vi "Initial Signal Processing.vi"(8 "error in":errorcluster, 11 "AI Ref In":T1) -> (0 "error out":errorcluster, 1 "max value":dbl, 2 "Wheeze?":bool[](array[boolean]), 3 "AI Ref Out 2":T1)   [LabVIEW 2019]
doc: "The myRIO Project template acquires acceleration data from the onboard accelerometer and displays the changes of acceleration values in a waveform chart."
uses:
  <vilib>/myRIO/Instrument Drivers/Onboard IO/AI/typedefs/AI Reference.ctl
  <vilib>/myRIO/Common/Instrument Driver Framework/Utilities/typedefs/myRIO Generic Hardware Reference.ctl
  <vilib>/myRIO/Common/Instrument Driver Framework/Utilities/typedefs/Hardware Version Enum.ctl
  <vilib>/myRIO/Common/Instrument Driver Framework/Utilities/typedefs/myRIO v1.0 Reference.ctl
  <vilib>/myRIO/Common/Instrument Driver Framework/Utilities/typedefs/Generic FPGA Reference.ctl
  <vilib>/myRIO/Common/Instrument Driver Framework/myRIO v1.0/AI/typedefs/AI Channels List.ctl
  <vilib>/myRIO/Common/Instrument Driver Framework/myRIO v1.0/AI/typedefs/AI Channels Enum.ctl
  <vilib>/myRIO/Common/Instrument Driver Framework/Utilities/typedefs/Analog Scaling Constants List.ctl
  <vilib>/myRIO/Common/Instrument Driver Framework/Utilities/typedefs/Analog Scaling Constants.ctl
  <vilib>/Platform/TimedLoop/XDataNode/timing_clust.ctl
  <vilib>/Platform/TimedLoop/XDataNode/nitl_modes.ctl
  <vilib>/Platform/TimedLoop/XDataNode/wakeup.ctl
  <vilib>/Analysis/baseanly.llb/Mean (DBL).vi
  <vilib>/Utility/error.llb/Error Cluster From Error Code.vi
  <vilib>/myRIO/Common/Instrument Driver Framework/myRIO v1.0/AI/vis/myRIO v1.0 Read AI.vi
  <vilib>/platform/TimedLoop/XDataNode/XDataNode.xnode
  <vilib>/Platform/TimedLoop/XDataNode/XDNodeRunTimeDep.lvlib
  <vilib>/myRIO/Instrument Drivers/Onboard IO/AI/AI.lvlib
  <vilib>/Analysis/NI_AALBase.lvlib
panel:
  out "AI Ref Out 3":T1
  in  "AI Ref In 2":T1
  out "Waveform Chart":dbl[](graph)
  out "x-y":dbl[](array[numeric])
  in  "[ESC]":bool
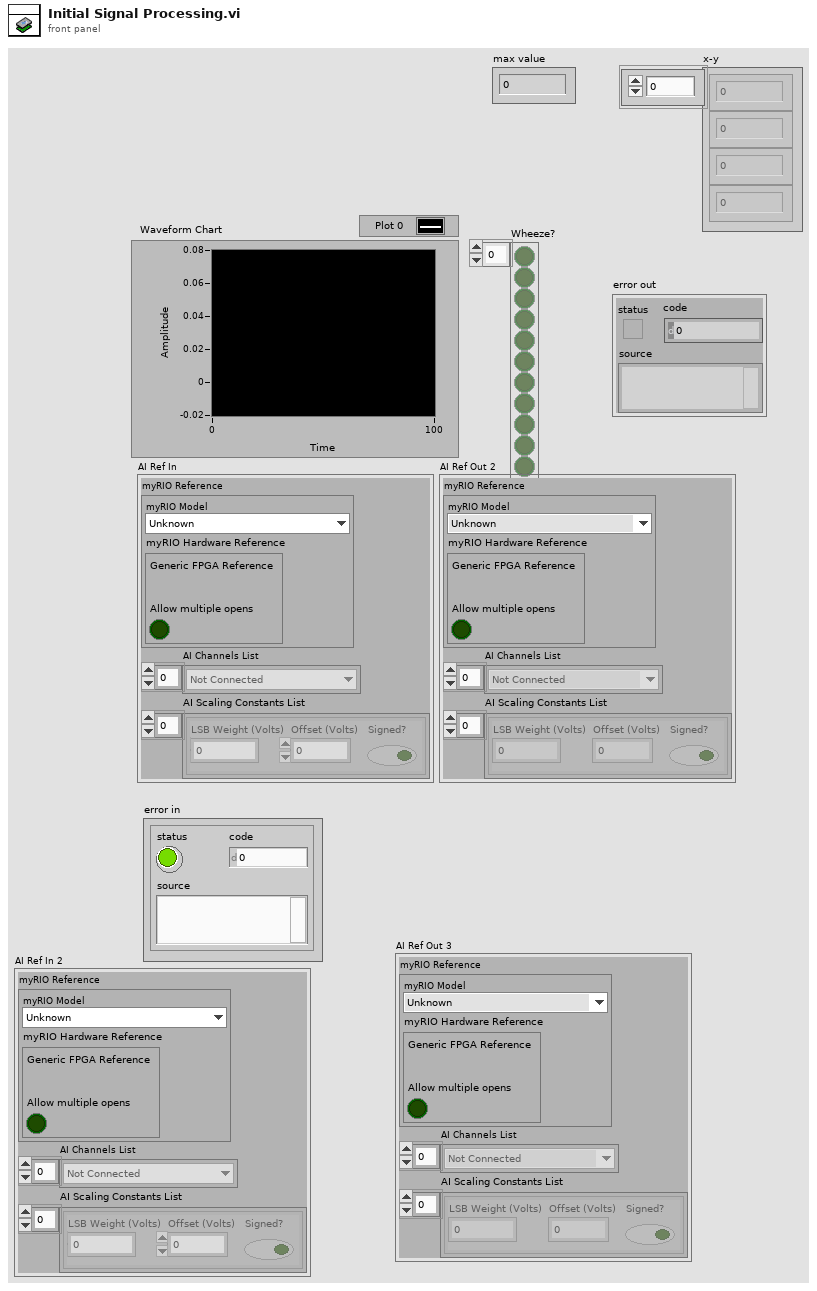
[diagram p1: front panel]
types:
  T1 = typedef "AI.lvlib/AI Reference.ctl" = cluster{"myRIO Reference":T2, "AI Channels List":T6, "AI Scaling Constants List":T8}
  T2 = typedef "myRIO Generic Hardware Reference.ctl" = cluster{"myRIO Model":T3, "myRIO Hardware Reference":T4}
  T3 = typedef "Hardware Version Enum.ctl" = enum16{"Unknown", "myRIO-1900", "myRIO-1950", "roboRIO", "NI ELVIS RIO CM", "ELVIS III"}
  T4 = typedef "myRIO v1.0 Reference.ctl" = cluster{"Generic FPGA Reference":T5, "Allow multiple opens":bool}
  T5 = typedef "Generic FPGA Reference.ctl" = refnum<k20>
  T6 = typedef "AI Channels List.ctl" = T7[]
  T7 = typedef "AI Channels Enum.ctl" = enum16{"Not Connected", "AudioIn/Left", "AudioIn/Right", "C/AI0", "C/AI1", "A/AI0", "A/AI1", "A/AI2", "A/AI3", "A/AI4", "A/AI5", "A/AI6", "A/AI7", "B/AI0", "B/AI1", "B/AI2", "B/AI3", "B/AI4", "B/AI5", "B/AI6", "B/AI7", "AI/AI0", "AI/AI1", "AI/AI2", "AI/AI3", "A/AI0 (DIFF)", "A/AI1 (DIFF)", "A/AI2 (DIFF)", "A/AI3 (DIFF)", "B/AI0 (DIFF)", "B/AI1 (DIFF)", "B/AI2 (DIFF)", "B/AI3 (DIFF)"}
  T8 = typedef "Analog Scaling Constants List.ctl" = T9[]
  T9 = typedef "Analog Scaling Constants.ctl" = cluster{"LSB Weight (Volts)":dbl, "Offset (Volts)":dbl, "Signed?":bool}
  T10 = typedef "XDNodeRunTimeDep.lvlib/timing_clust.ctl" = cluster{"Expected End [f-1]":u64, "Actual End [f-1]":u64, "Finished Late? [f-1]":bool, "Expected End [i-1]":u64, "Actual End [i-1]":u64, "Finished Late? [i-1]":bool, "Expected Start [i]":u64, "Actual Start [i]":u64, "Expected Start [f]":u64, "Actual Start [f]":u64, "Source Name":string, "Structure Name":string, "Period":i64, "Deadline":i64, "Offset":i64, "Start":i64, "Priority":i32, "Timeout":i32, "Mode":T11, "Wakeup Reason":T12, "Error":errorcluster, "Source Type":string, "Secondary Source Type":string, "Global End Time":u64, "Global Start Time":u64, "Frame Duration":u64, "Iteration Duration":u64, "Assigned CPU":i32, "I/O Scan Engine Mode":u32}
  T11 = typedef "XDNodeRunTimeDep.lvlib/nitl_modes.ctl" = enum32{"No Change", "Process missed periods, maintain original phase", "Discard missed periods, maintain original phase", "Process missed periods, ignore original phase", "Discard missed periods, ignore original phase"}
  T12 = typedef "XDNodeRunTimeDep.lvlib/wakeup.ctl" = enum32{"Normal", "Aborted", "Asynchronous wakeup", "Timing source error", "Timed loop error", "Timeout"}
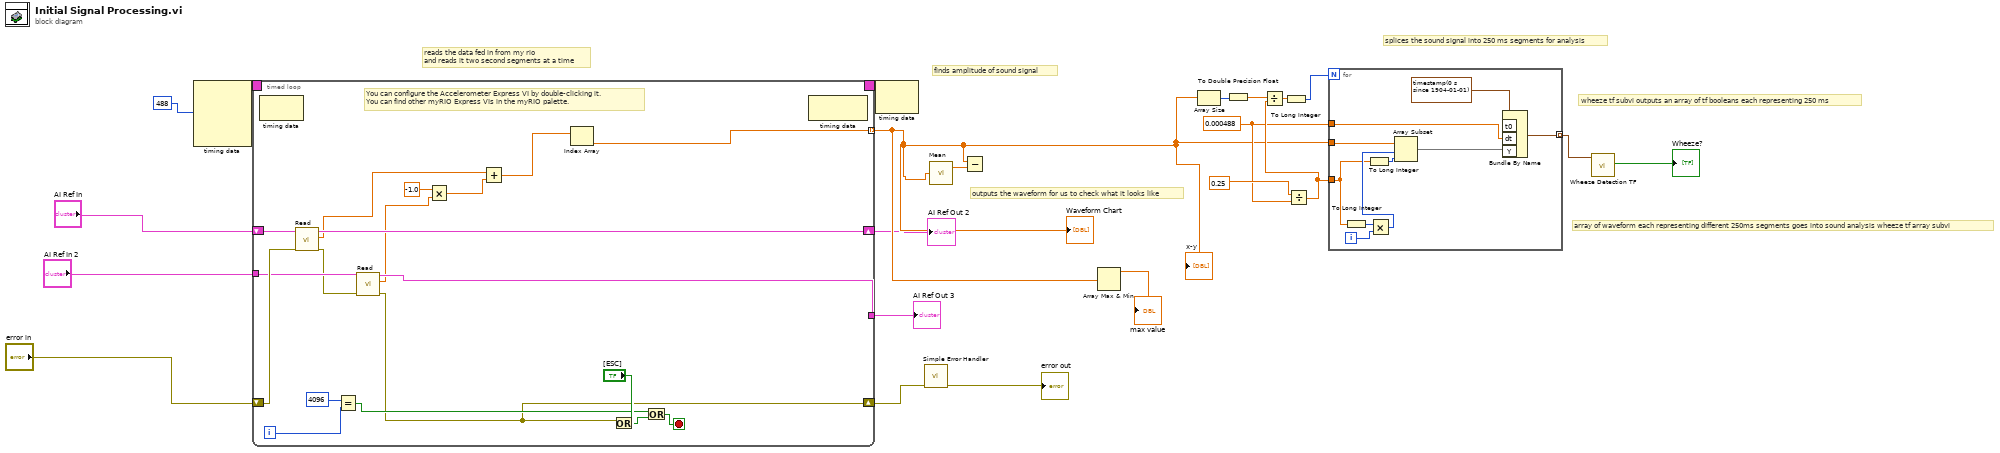
[diagram p0: block diagram]
diagram:
  w8 = 0.000488 ("dt")
  # "wheeze tf subvi outputs an array of tf booleans each representing 250 ms"
  # "array of waveform each representing different 250ms segments goes into sound analysis wheeze tf array subvi"
  # "splices the sound signal into 250 ms segments for analysis"
  # "outputs the waveform for us to check what it looks like"
  # "finds amplitude of sound signal"
  # "reads the data fed in from my rio\nand reads it two second segments at a time"
  # "You can configure the Accelerometer Express VI by double-clicking it.\nYou can find other myRIO Express VIs in the myRIO palette."
  n1 = node-c288(i64 488 ("Period")) -> (w22:T10)  [unwired: 3 in]
  n2 = timed-loop {
    timing: w22 -> [_]
    timing-out: [_] -> w21
    tunnel: [w39] -> w7 mode=indexing
    shift-right: [w33] -> w3
    shift-left: "AI Ref In" -> [w40]
    shift-right: [w28] -> w19
    shift-left: "error in" -> [w32]
    tunnel: "AI Ref In 2" -> [w31]
    tunnel: [w30] -> w1
    i -> [w38]
    stop <- w34 stop-if-true
    n3 = node-c288() -> ()  [unwired: 1 in, 1 out]
    n4 = call <vilib>:"Read.vi"("error in (no error)"=w32, "AI Ref In"=w40) -> ("error out"=w29:errorcluster, "Values"=w24:dbl[], "AI Ref Out"=w33:T1)  [unwired: 7 in]
    n5 = Equal?(x=4096, y=w38) -> (x = y?=w36:bool)
    n6 = call <vilib>:"Read.vi"("error in (no error)"=w29, "AI Ref In"=w31) -> ("error out"=w28:errorcluster, "Values"=w26:dbl[], "AI Ref Out"=w30:T1)  [unwired: 7 in]
    n7 = Multiply(x=-1.0, y=w26) -> (x*y=w25:dbl[])
    n8 = Add(x=w24, y=w25) -> (x+y=w23:dbl[])
    n9 = Index Array "Index Array"(array=w23) -> (element=w39:dbl)  [unwired: 1 in]
    n10 = Or(x=w28, y="[ESC]") -> (x .or. y?=w35:bool)
    n11 = Or(x=w36, y=w35) -> (x .or. y?=w34:bool)
    n12 = node-c288() -> ()  [unwired: 1 in, 1 out]
  }
  "x-y" <- w7
  "Waveform Chart" <- w7
  "AI Ref Out 2" <- w3
  "AI Ref Out 3" <- w1
  n13 = node-c288(w21) -> ()  [unwired: 1 out]
  n14 = call <vilib>:"Simple Error Handler.vi"("error in (no error)"=w19) -> ("error out"=→"error out":errorcluster)  [unwired: 4 in, 4 out]
  n15 = call-poly <vilib>:"Mean.vi"("X"=w7) -> ("mean"=w17:dbl)  [unwired: 1 out]
  n16 = Subtract(x=w7, y=w17) -> ()  [unwired: 1 out]
  n17 = Array Max & Min(array=w7) -> (max value=→"max value":dbl)  [unwired: 3 out]
  n18 = Array Size(array=w7) -> (size(s)=w14:i32)
  n19 = To Double Precision Float(number=w14) -> (double precision float=w13:dbl)
  n20 = Divide(x=0.25 ("y"), y=w8) -> (x/y=w10:dbl)
  n21 = Divide(x=w13, y=w10) -> (x/y=w12:dbl)
  n22 = To Long Integer(number=w12) -> (32bit integer=w11:i32)
  n23 = for {
    N: w11 -> [_]
    tunnel: [w52] -> w15 mode=indexing
    tunnel: w7 -> [w51]
    tunnel: w10 -> [w45]
    tunnel: w8 -> [w44]
    i -> [w49]
    n24 = To Long Integer(number=w45) -> (32bit integer=w47:i32)
    n25 = To Long Integer(number=w45) -> (32bit integer=w46:i32)
    n26 = Multiply(x=w47, y=w49) -> (x*y=w48:i32)
    n27 = Array Subset(array=w51, index=w48, length=w46) -> (w50:dbl[])
    n28 = Bundle By Name("t0"=timestamp(0 s since 1904-01-01), "dt"=w44, "Y"=w50) -> (w52:waveform(dbl))  [unwired: 1 in]
  }
  n29 = call "Wheeze Detection TF.vi"("Array 2"=w15) -> ("Array"=→"Wheeze?":bool[])  [unwired: 10 in]
